vi "RP write file.vi"(5 "I-V avg":i32=480, 6 "Signal bits":i32=14, 7 "Mode":T2=enum."Digitizer", 8 "Error In":errorcluster, 9 "Channel info":T1[](array[typedef]) {"waveform start" format="%#_6p"; "waveform period" format="%#_6p"}, 10 "Data":string, 11 "File Path":path) -> (0 "Error Out":errorcluster, 1 "Channel names":string[](array[string]), 3 "File  path out":path)   [LabVIEW 2016]
uses:
  Mode.ctl
  RP info.ctl
  <vilib>/Utility/tdmsutil.llb/TDMS Create Scaling Information (Linear).vi
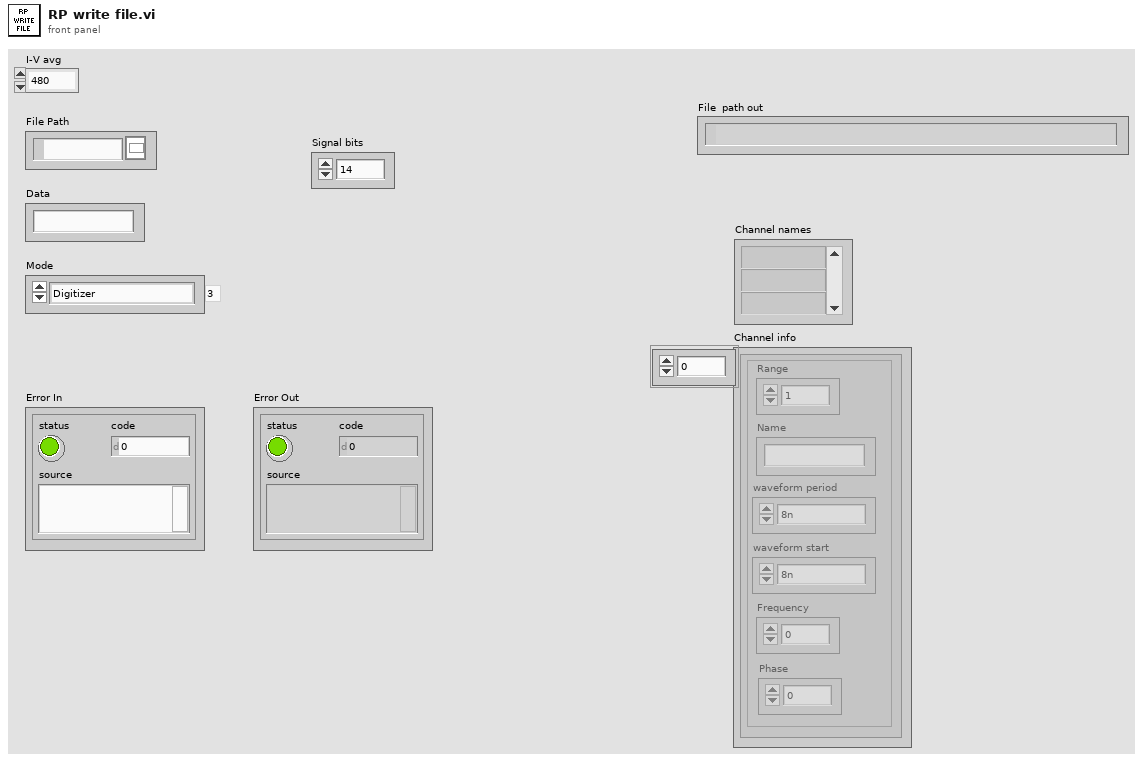
[diagram p1: front panel]
types:
  T1 = typedef "RP info.ctl" = cluster{"Range":dbl, "Name":string, "waveform period":dbl, "waveform start":dbl, "Frequency":u32, "Phase":u32}
  T2 = typedef "Mode.ctl" = enum16{"Filter", "Lockin test", "Snapshot test", "Digitizer", "Current-Voltage"}
  T3 = enum16{"open", "open or create", "create or replace", "create", "open (read-only)"}
  T4 = enum16{"big-endian, network order", "native, host order", "little-endian"}
  T5 = cluster{"slope":dbl, "y intercept":dbl, "input source":i32}
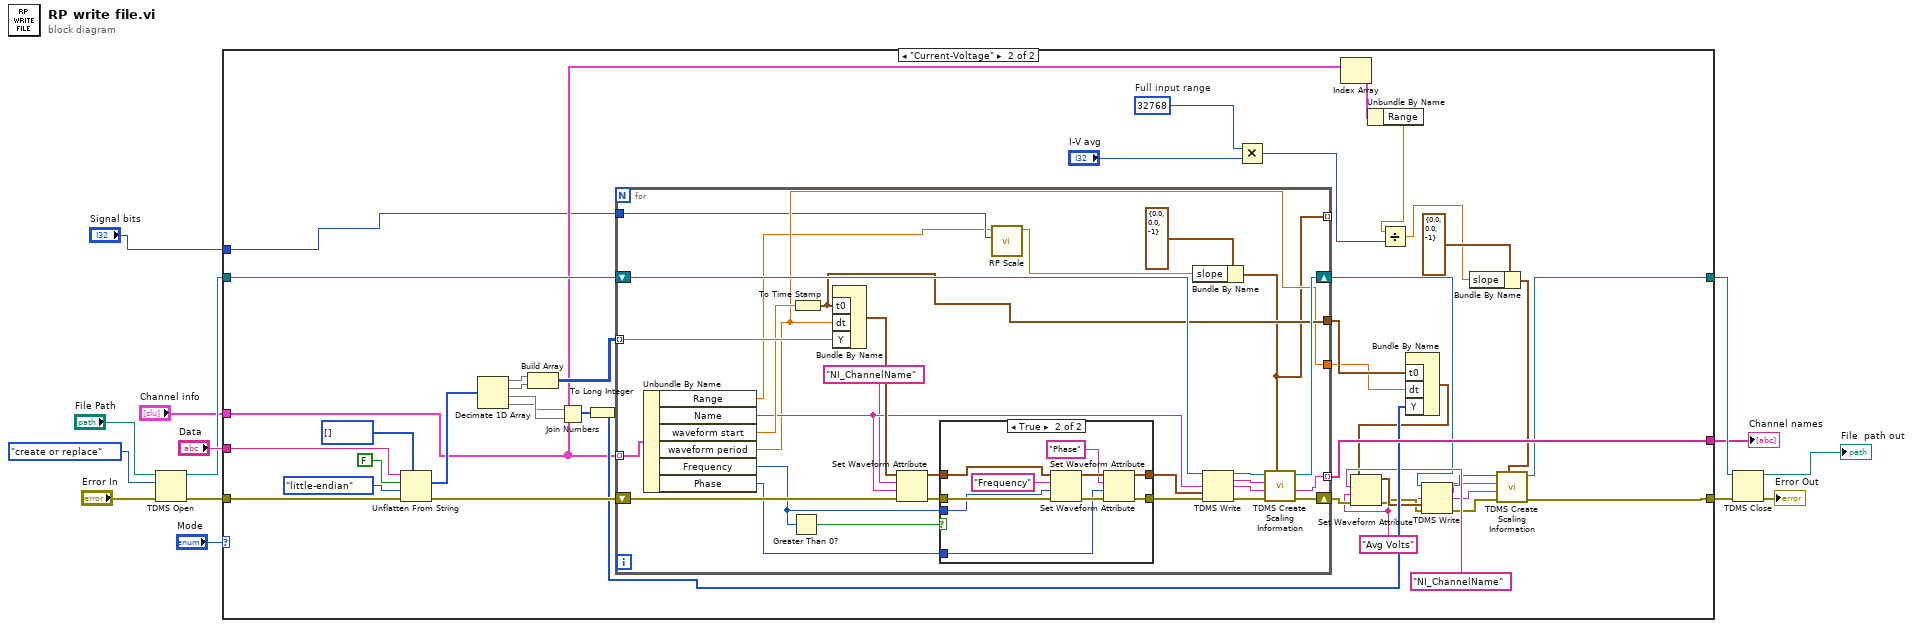
[diagram p0: block diagram]
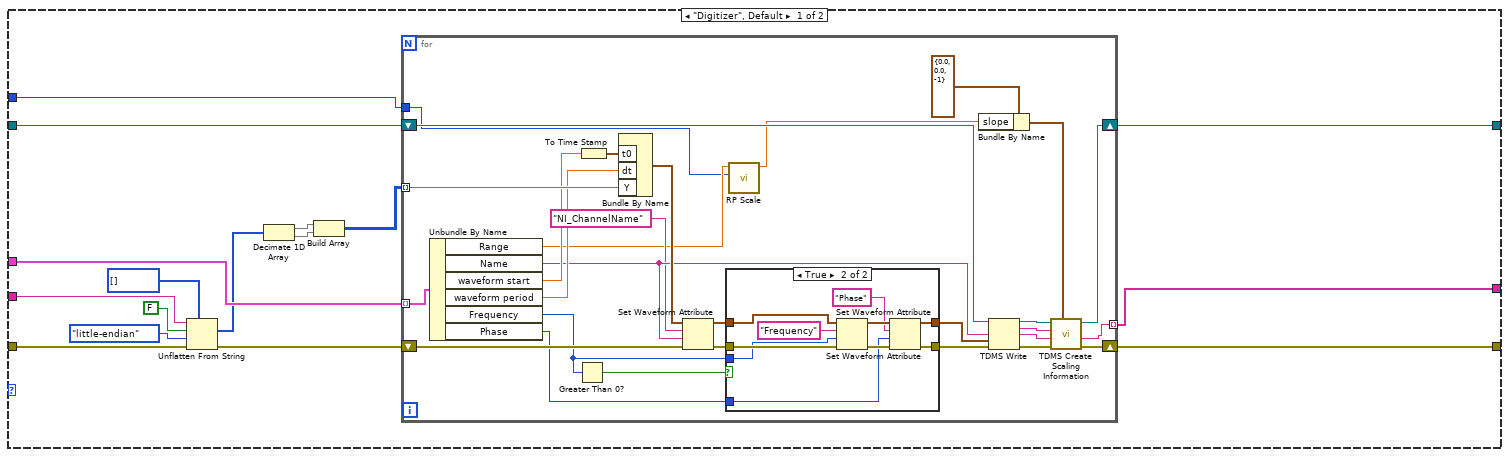
[diagram p2: hidden frame]
diagram:
  n1 = TDMS Open(8:"Error In", 10:T3."create or replace" ("operation (0:open)"), 11:"File Path") -> (0:w9:errorcluster, 3:w8:refnum<k34>)  [unwired: 4 in]
  n2 = case shown="\"Current-Voltage\"" "Mode" {
    tunnel: "Data" -> [w28 w110]
    tunnel: w9 -> [w27 w109]
    tunnel: w8 -> [w23 w106]
    tunnel: "Channel info" -> [w25 w79]
    tunnel: [w22 w85] -> w6
    tunnel: [w21 w87] -> w5
    tunnel: "Signal bits" -> [w15 w72]
    tunnel: [w16 w101] -> w2
    frame "Digitizer", Default {
      n3 = Unflatten From String(type=i16[] [], binary string=w28, data includes array or string size? (T)=FALSE, byte order (0:big-endian, network order)=T4."little-endian", error in (no error)=w27) -> (value=w20:i16[], error out=w24:errorcluster)  [unwired: 1 out]
      n4 = Decimate 1D Array(w20) -> (w19:i16[], w18:i16[])
      n5 = Build Array(w19, w18) -> (w17:i16[][])
      n6 = for {
        tunnel: w17 -> [w58] mode=indexing
        tunnel: w25 -> [w59] mode=indexing
        shift-right: [w45] -> w22
        shift-left: w24 -> [w42]
        shift-right: [w51] -> w21
        shift-left: w23 -> [w54]
        tunnel: [w34] -> w16 mode=indexing
        tunnel: w15 -> [w32]
        n7 = Unbundle By Name(w59) -> ("Range"=w33:dbl, "Name"=w43:string, "waveform start"=w55:dbl, "waveform period"=w57:dbl, "Frequency"=w36:u32, "Phase"=w35:u32)
        n8 = Greater Than 0?(x=w36) -> (x > 0?=w37:bool)
        n9 = To Time Stamp(1:w55) -> (0:w56:timestamp)
        n10 = Bundle By Name("t0"=w56, "dt"=w57, "Y"=w58) -> (w52:waveform(i16))  [unwired: 1 in]
        n11 = Set Waveform Attribute(4:w42, 5:w43, 6:"NI_ChannelName" ("name"), 7:w52) -> (0:w38:errorcluster, 3:w44:waveform(i16))  [unwired: 1 out]
        n12 = case shown="True" w37 {
          tunnel: w44 -> [w60 w71]
          tunnel: [w60 w69] -> w40
          tunnel: [w61 w68] -> w39
          tunnel: w38 -> [w61 w67]
          tunnel: w36 -> [_ w64]
          tunnel: w35 -> [_ w62]
          frame False {
          }
          frame True {
            n13 = Set Waveform Attribute(4:w67, 5:w64, 6:"Frequency" ("name"), 7:w71) -> (0:w66:errorcluster, 3:w70:waveform(i16))  [unwired: 1 out]
            n14 = Set Waveform Attribute(4:w66, 5:w62, 6:"Phase" ("name"), 7:w70) -> (0:w68:errorcluster, 3:w69:waveform(i16))  [unwired: 1 out]
          }
        }
        n15 = call "RP Scale.vi"("Signal bits"=w32, "Range"=w33) -> ("Slope"=w31:dbl)  [unwired: 7 in, 2 out]
        n16 = Bundle By Name(cluster=T5 {"slope"=0.0, "y intercept"=0.0, "input source"=-1} ("linear scale"), "slope"=w31) -> (w46:T5)
        n17 = TDMS Write(0:w54, 7:w43, 9:w40, 11:w39) -> (4:w53:refnum<k34>, 6:w49:string, 8:w48:string, 15:w50:errorcluster)  [unwired: 2 in]
        n18 = call-poly <vilib>:"TDMS Create Scaling Information.vi"("linear scale"=w46, "error in (no error)"=w50, "channel name"=w48, "group name"=w49, "tdms file"=w53) -> ("error out"=w45:errorcluster, "channel name out"=w34:string, "tdms file out"=w51:refnum<k34>)  [unwired: 2 in, 2 out]
      }
    }
    frame "Current-Voltage" {
      w76 = 32768  # Full input range
      w82 = "Avg Volts"
      n19 = Unflatten From String(type=i16[] [], binary string=w110, data includes array or string size? (T)=FALSE, byte order (0:big-endian, network order)=T4."little-endian", error in (no error)=w109) -> (value=w105:i16[], error out=w107:errorcluster)  [unwired: 1 out]
      n20 = Decimate 1D Array(w105) -> (w104:i16[], w103:i16[], w100:i16[], w99:i16[])
      n21 = Build Array(w104, w103) -> (w102:i16[][])
      n22 = Join Numbers(hi=w99, lo=w100) -> ((hi.lo)=w98:u32[])
      n23 = To Long Integer(number=w98) -> (32bit integer=w97:i32[])
      n24 = for {
        tunnel: w102 -> [w140] mode=indexing
        tunnel: w79 -> [w141] mode=indexing
        shift-right: [w130] -> w94
        shift-left: w107 -> [w127]
        shift-right: [w135] -> w88
        shift-left: w106 -> [w138]
        tunnel: [w119] -> w101 mode=indexing
        tunnel: [w118] -> w96
        tunnel: [w117] -> w95
        tunnel: [w116] -> _ mode=indexing
        tunnel: w72 -> [w115]
        n25 = Unbundle By Name(w141) -> ("Range"=w114:dbl, "Name"=w128:string, "waveform start"=w139:dbl, "waveform period"=w117:dbl, "Frequency"=w121:u32, "Phase"=w120:u32)
        n26 = Greater Than 0?(x=w121) -> (x > 0?=w122:bool)
        n27 = To Time Stamp(1:w139) -> (0:w118:timestamp)
        n28 = Bundle By Name("t0"=w118, "dt"=w117, "Y"=w140) -> (w136:waveform(i16))  [unwired: 1 in]
        n29 = Set Waveform Attribute(4:w127, 5:w128, 6:"NI_ChannelName" ("name"), 7:w136) -> (0:w123:errorcluster, 3:w129:waveform(i16))  [unwired: 1 out]
        n30 = case shown="True" w122 {
          tunnel: w129 -> [w142 w153]
          tunnel: [w142 w151] -> w125
          tunnel: [w143 w150] -> w124
          tunnel: w123 -> [w143 w149]
          tunnel: w121 -> [_ w146]
          tunnel: w120 -> [_ w144]
          frame False {
          }
          frame True {
            n31 = Set Waveform Attribute(4:w149, 5:w146, 6:"Frequency" ("name"), 7:w153) -> (0:w148:errorcluster, 3:w152:waveform(i16))  [unwired: 1 out]
            n32 = Set Waveform Attribute(4:w148, 5:w144, 6:"Phase" ("name"), 7:w152) -> (0:w150:errorcluster, 3:w151:waveform(i16))  [unwired: 1 out]
          }
        }
        n33 = call "RP Scale.vi"("Signal bits"=w115, "Range"=w114) -> ("Slope"=w113:dbl)  [unwired: 7 in, 2 out]
        n34 = Bundle By Name(cluster=T5 {"slope"=0.0, "y intercept"=0.0, "input source"=-1} ("linear scale"), "slope"=w113) -> (w116:T5)
        n35 = TDMS Write(0:w138, 7:w128, 9:w125, 11:w124) -> (4:w137:refnum<k34>, 6:w133:string, 8:w132:string, 15:w134:errorcluster)  [unwired: 2 in]
        n36 = call-poly <vilib>:"TDMS Create Scaling Information.vi"("linear scale"=w116, "error in (no error)"=w134, "channel name"=w132, "group name"=w133, "tdms file"=w137) -> ("error out"=w130:errorcluster, "channel name out"=w119:string, "tdms file out"=w135:refnum<k34>)  [unwired: 2 in, 2 out]
      }
      n37 = Multiply(x=w76, y="I-V avg") -> (x*y=w74:i32)
      n38 = Index Array(array=w79) -> (element=w78:T1)  [unwired: 1 in]
      n39 = Unbundle By Name(w78) -> ("Range"=w77:dbl)
      n40 = Divide(x=w77, y=w74) -> (x/y=w80:dbl)
      n41 = Bundle By Name("t0"=w96, "dt"=w95, "Y"=w97) -> (w92:waveform(i32))  [unwired: 1 in]
      n42 = Set Waveform Attribute(4:w94, 5:w82, 6:"NI_ChannelName" ("name"), 7:w92) -> (0:w90:errorcluster, 3:w91:waveform(i32))  [unwired: 1 out]
      n43 = TDMS Write(0:w88, 7:w82, 9:w91, 11:w90) -> (4:w89:refnum<k34>, 6:w84:string, 8:w83:string, 15:w86:errorcluster)  [unwired: 2 in]
      n44 = Bundle By Name(cluster=T5 {"slope"=0.0, "y intercept"=0.0, "input source"=-1} ("linear scale"), "slope"=w80) -> (w73:T5)
      n45 = call-poly <vilib>:"TDMS Create Scaling Information.vi"("linear scale"=w73, "error in (no error)"=w86, "channel name"=w83, "group name"=w84, "tdms file"=w89) -> ("error out"=w85:errorcluster, "tdms file out"=w87:refnum<k34>)  [unwired: 2 in, 3 out]
    }
  }
  "Channel names" <- w2
  n46 = TDMS Close(8:w6, 11:w5) -> (0:→"Error Out":errorcluster, 3:→"File  path out":path)
